vi "ke2000 VI Tree.vi"   [LabVIEW 2010]
doc: "This is the instrument driver for the Keithley 2000 Series instruments. The VI Tree displays all the user-callable VIs of the instrument driver in an organized table.\n\nThis VI Tree contains all of the VI's in the LabVIEW template driver. These VI's are intended to be used as starting points for creating your own driver VIs for a particular instrument. Most of these VIs are not operational until they are modified. Rename and save them into your own .LLB file as you modify them for your instrument. ALL National Instrument drivers must include the VI's included in this VI Tree (Initialize, all utility VI's, and Close). You should place all non-user-callable VI's in a utility .LLB. An example of this is the CoreDr_U.LLB file, which contains the non-user-callable VI's for the template driver."
uses:
  <instrlib>/ke2000/ke2000.llb/ke2000 Configure Measurement.vi
  <instrlib>/ke2000/ke2000.llb/ke2000 Configure Route Single.vi
panel:
  # "SEE DIAGRAM\nFOR VI TREE."
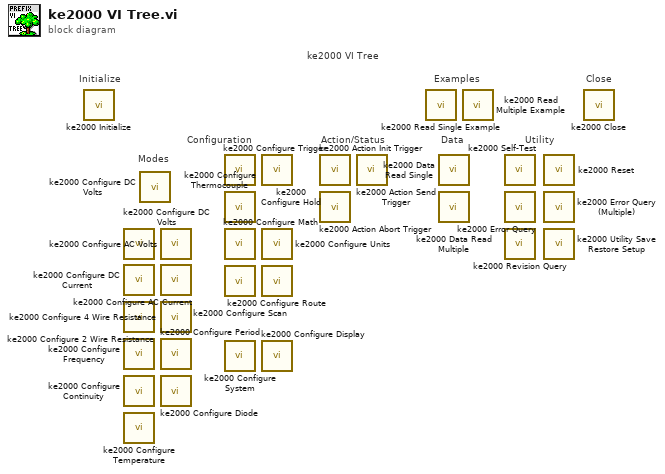
[diagram p0: block diagram]
diagram:
  # "Modes"
  # "ke2000 VI Tree"
  # "Examples"
  # "Configuration"
  # "Utility"
  # "Data"
  # "Action/Status"
  # "Close"
  # "Initialize"
  n1 = call <instrlib>:"ke2000 Initialize.vi"() -> ()  [unwired: 18 in, 2 out]
  n2 = call <instrlib>:"ke2000 Configure DC Volts.vi"() -> ()  [unwired: 18 in, 2 out]
  n3 = call <instrlib>:"ke2000 Configure DC Current.vi"() -> ()  [unwired: 18 in, 2 out]
  n4 = call <instrlib>:"ke2000 Configure 2 Wire Resistance.vi"() -> ()  [unwired: 18 in, 2 out]
  n5 = call <instrlib>:"ke2000 Configure Frequency.vi"() -> ()  [unwired: 18 in, 2 out]
  n6 = call <instrlib>:"ke2000 Configure Continuity.vi"() -> ()  [unwired: 18 in, 2 out]
  n7 = call <instrlib>:"ke2000 Configure Temperature.vi"() -> ()  [unwired: 18 in, 2 out]
  n8 = call-poly <instrlib>:"ke2000 Configure DC Volts.vi"() -> ()  [unwired: 18 in, 2 out]
  n9 = call <instrlib>:"ke2000 Configure AC Volts.vi"() -> ()  [unwired: 18 in, 2 out]
  n10 = call <instrlib>:"ke2000 Configure AC Current.vi"() -> ()  [unwired: 18 in, 2 out]
  n11 = call <instrlib>:"ke2000 Configure 4 Wire Resistance.vi"() -> ()  [unwired: 18 in, 2 out]
  n12 = call <instrlib>:"ke2000 Configure Period.vi"() -> ()  [unwired: 18 in, 2 out]
  n13 = call <instrlib>:"ke2000 Configure Diode.vi"() -> ()  [unwired: 18 in, 2 out]
  n14 = call <instrlib>:"ke2000 Configure Trigger.vi"() -> ()  [unwired: 18 in, 2 out]
  n15 = call <instrlib>:"ke2000 Configure Thermocouple.vi"() -> ()  [unwired: 18 in, 2 out]
  n16 = call <instrlib>:"ke2000 Configure Math.vi"() -> ()  [unwired: 18 in, 2 out]
  n17 = call <instrlib>:"ke2000 Configure Scan.vi"() -> ()  [unwired: 18 in, 2 out]
  n18 = call <instrlib>:"ke2000 Configure System.vi"() -> ()  [unwired: 18 in, 2 out]
  n19 = call <instrlib>:"ke2000 Configure Hold.vi"() -> ()  [unwired: 18 in, 2 out]
  n20 = call <instrlib>:"ke2000 Configure Units.vi"() -> ()  [unwired: 18 in, 2 out]
  n21 = call-poly <instrlib>:"ke2000 Configure Route.vi"() -> ()  [unwired: 18 in, 2 out]
  n22 = call <instrlib>:"ke2000 Configure Display.vi"() -> ()  [unwired: 18 in, 2 out]
  n23 = call <instrlib>:"ke2000 Action Init Trigger.vi"() -> ()  [unwired: 18 in, 2 out]
  n24 = call <instrlib>:"ke2000 Action Abort Trigger.vi"() -> ()  [unwired: 18 in, 2 out]
  n25 = call <instrlib>:"ke2000 Action Send Trigger.vi"() -> ()  [unwired: 18 in, 2 out]
  n26 = call <instrlib>:"ke2000 Read Single Example.vi"() -> ()  [unwired: 20 in]
  n27 = call <instrlib>:"ke2000 Data Read Single.vi"() -> ()  [unwired: 15 in, 5 out]
  n28 = call <instrlib>:"ke2000 Data Read Multiple.vi"() -> ()  [unwired: 15 in, 5 out]
  n29 = call <instrlib>:"ke2000 Read Multiple Example.vi"() -> ()  [unwired: 20 in]
  n30 = call <instrlib>:"ke2000 Self-Test.vi"() -> ()  [unwired: 16 in, 4 out]
  n31 = call <instrlib>:"ke2000 Error Query.vi"() -> ()  [unwired: 16 in, 4 out]
  n32 = call <instrlib>:"ke2000 Revision Query.vi"() -> ()  [unwired: 16 in, 4 out]
  n33 = call <instrlib>:"ke2000 Reset.vi"() -> ()  [unwired: 18 in, 2 out]
  n34 = call <instrlib>:"ke2000 Error Query (Multiple).vi"() -> ()  [unwired: 17 in, 3 out]
  n35 = call <instrlib>:"ke2000 Utility Save Restore Setup.vi"() -> ()  [unwired: 18 in, 2 out]
  n36 = call <instrlib>:"ke2000 Close.vi"() -> ()  [unwired: 19 in, 1 out]
